vi "MinimumJerkGenerateNext.vi"(8 "error in (no error)":errorcluster, 10 "Target y":dbl, 11 "Target x":dbl) -> (0 "error out":errorcluster, 2 "yt":dbl, 3 "xt":dbl)   [LabVIEW 2017, in "admittanceControllerLibrary.lvlib"]
uses:
  admittanceControllerLibrary.lvlib
  Controls/initial conditions control.ctl
  Controls/timer control.ctl
  Controls/tf control.ctl
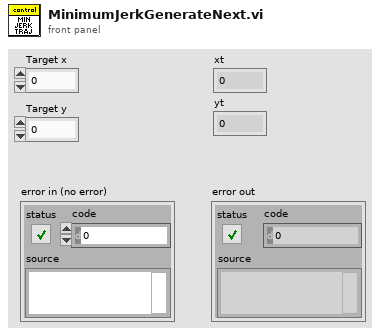
[diagram p1: front panel]
types:
  T1 = typedef "admittanceControllerLibrary.lvlib/tf control.ctl" = enum16{"get tf", "set tf"}
  T2 = typedef "admittanceControllerLibrary.lvlib/timer control.ctl" = enum16{"get time", "set time"}
  T3 = typedef "admittanceControllerLibrary.lvlib/initial conditions control.ctl" = enum16{"get", "set"}
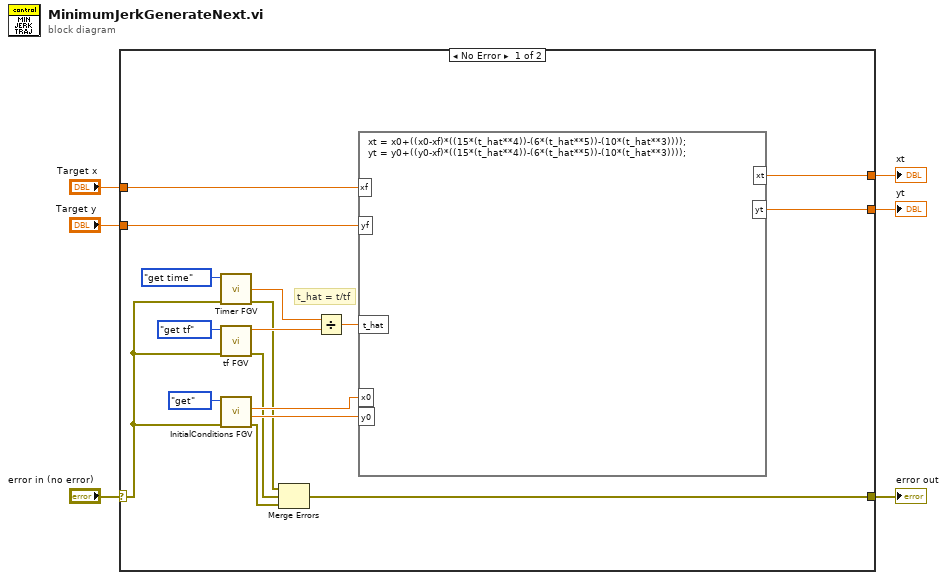
[diagram p0: block diagram]
diagram:
  n1 = case shown="No Error" "error in (no error)" {
    selector: "error in (no error)" -> [w11 w24]
    tunnel: "Target x" -> [w23 _]
    tunnel: "Target y" -> [w22 _]
    tunnel: [w20 _] -> w4
    tunnel: [w19 _] -> w3
    tunnel: [w7 w24] -> w1
    frame No Error {
      # "t_hat = t/tf"
      n2 = call "Timer FGV.vi"("error in (no error)"=w11, "Enum"=timer_control."get time") -> ("error out"=w10:errorcluster, "Elapsed Time"=w13:dbl)  [unwired: 8 in]
      n3 = call "tf FGV.vi"("error in (no error)"=w11, "Enum"=tf_control."get tf") -> ("error out"=w9:errorcluster, "tf"=w12:dbl)  [unwired: 8 in]
      n4 = call "InitialConditions FGV.vi"("error in (no error)"=w11, "Enum"=initial_conditions_control."get") -> ("error out"=w8:errorcluster, "Y0"=w16:dbl, "X0"=w17:dbl)  [unwired: 7 in]
      n5 = Merge Errors(w10, w9, w8) -> (w7:errorcluster)
      n6 = Divide(x=w13, y=w12) -> (x/y=w21:dbl)
      n7 = formula code="xt = x0+((x0-xf)*((15*(t_hat**4))-(6*(t_hat**5))-(10*(t_hat**3))));\nyt = y0+((y0-xf)*((15*(t_hat**4))-(6*(t_hat**5))-(10*(t_hat**3))));"("t_hat"=w21, "x0"=w17, "y0"=w16, "xf"=w23, "yf"=w22) -> ("xt"=w20:dbl, "yt"=w19:dbl)
    }
    frame Error {
    }
  }
  "xt" <- w4
  "yt" <- w3
  "error out" <- w1
